vi "Show ErrorMesg.vi"(4 "error in (no error)":errorcluster) -> (0 "error out":errorcluster)   [LabVIEW 2023]
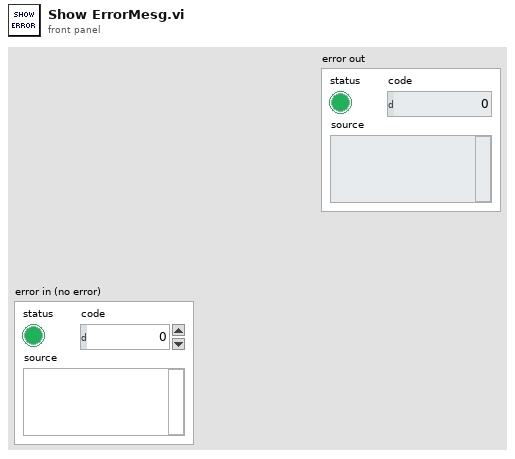
[diagram p1: front panel]
types:
  T1 = cluster{"status":bool, "code":bool, "source":bool}
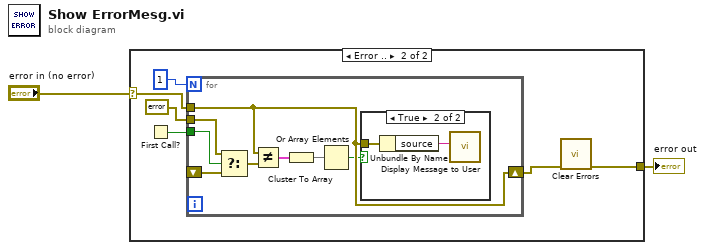
[diagram p0: block diagram]
diagram:
  n1 = case shown="Error .." "error in (no error)" {
    selector: "error in (no error)" -> [w3 w9]
    tunnel: [w3 w4] -> w1
    frame No Error {
    }
    frame Error {
      n2 = First Call?() -> (First Call?: T/F=w7:bool)
      n3 = for {
        N: 1 -> [_]
        tunnel: w9 -> [w17]
        shift-right: [w17] -> w5
        shift-left: _ -> [w11]
        tunnel: w7 -> [w13]
        tunnel: errorcluster {"status"=FALSE, "code"=0, "source"=""} ("error constant") -> [w12]
        n4 = Select(t=w12, s=w13, f=w11) -> (s? t:f=w10:errorcluster)
        n5 = Not Equal?(x=w17, y=w10) -> (x != y?=w16:T1)
        n6 = Cluster To Array(cluster=w16) -> (array=w15:bool[])
        n7 = Or Array Elements(Boolean array=w15) -> (logical OR=w14:bool)
        n8 = case shown="True" w14 {
          tunnel: w17 -> [_ w18]
          frame False {
          }
          frame True {
            n9 = Unbundle By Name(w18) -> ("source"=w19:string)
            n10 = call "Display Message to User"("Message"=w19) -> ()  [unwired: 9 in, 2 out]
          }
        }
      }
      n11 = call <vilib>:"Clear Errors.vi"("error in (no error)"=w5) -> ("error out"=w4:errorcluster)  [unwired: 5 in, 1 out]
    }
  }
  "error out" <- w1
